vi "Ejercicio_14_daq_sensor.vi"() -> ()   [LabVIEW 2020]
panel:
  out "XY Graph":cluster{dbl[], dbl[]}[](graph)
  out "Waveform Chart":dynamicdata(graph)
  out "array":dbl[](array[numeric])
  out "array 2":dbl[](array[numeric])
  in  "stop":bool
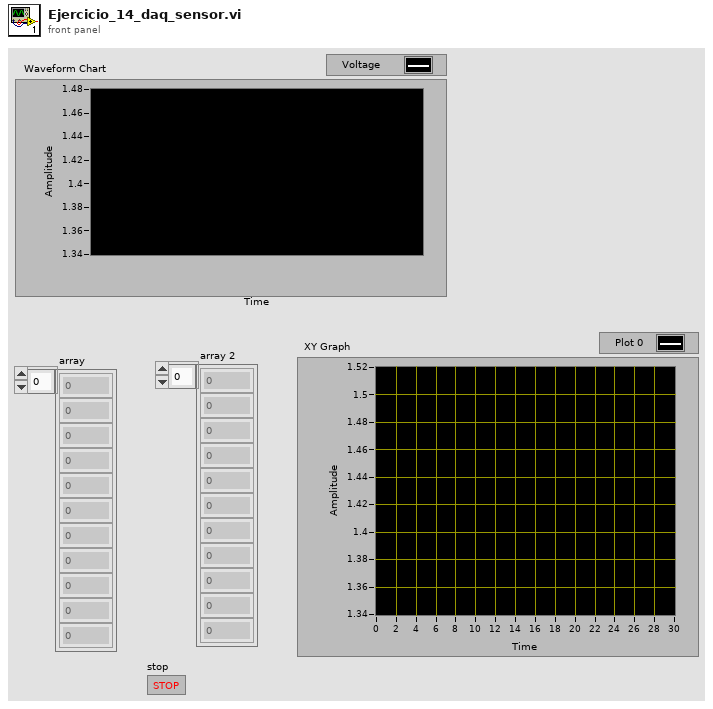
[diagram p1: front panel]
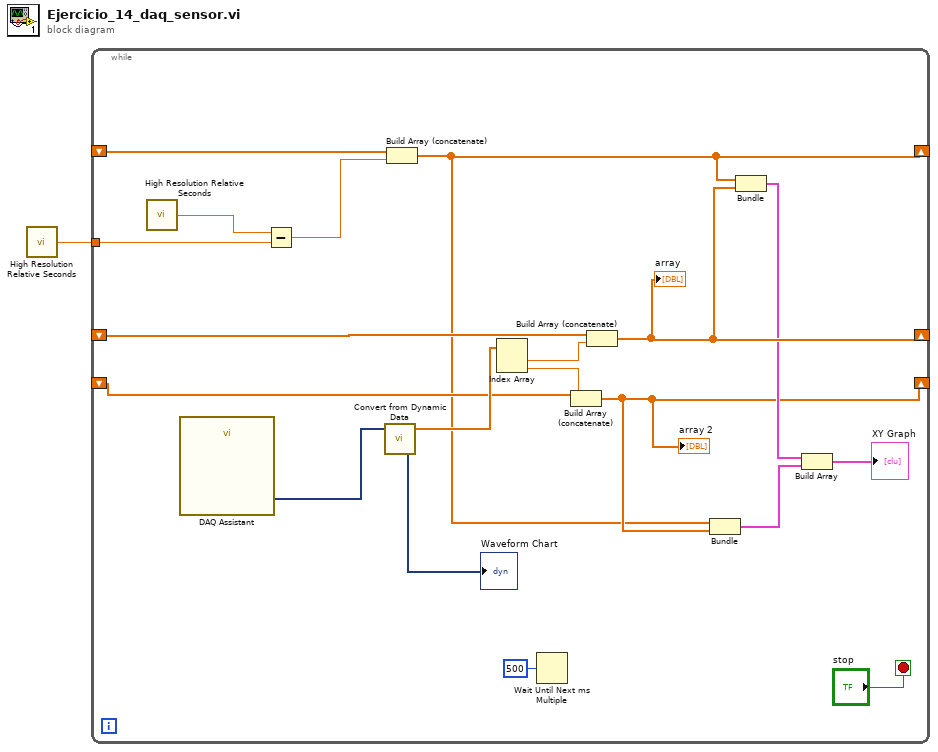
[diagram p0: block diagram]
diagram:
  n1 = call <vilib>:"High Resolution Relative Seconds.vi"() -> ("relative seconds"=w1:dbl)
  n2 = while {
    shift-right: [w8] -> _
    shift-left: _ -> [w15]
    shift-right: [w6] -> _
    shift-left: _ -> [w14]
    tunnel: w1 -> [w11]
    shift-right: [w5] -> _
    shift-left: _ -> [w9]
    stop <- "stop" stop-if-true
    n3 = call <vilib>:"High Resolution Relative Seconds.vi"() -> ("relative seconds"=w12:dbl)
    n4 = call "DAQ Assistant"() -> ("data"=w13:dynamicdata)  [unwired: 17 in, 2 out]
    "Waveform Chart" <- w13
    n5 = Subtract(x=w12, y=w11) -> (x-y=w10:dbl)
    n6 = call "Convert from Dynamic Data"("Dynamic Data Type"=w13) -> ("Array"=w18:dbl[])  [unwired: 3 in]
    n7 = Build Array (concatenate) "Build Array"(w9, w10) -> (w5:dbl[])
    n8 = Index Array "Index Array"(array=w18) -> (element #1=w16:dbl, element #2=w17:dbl)  [unwired: 2 in]
    n9 = Wait Until Next ms Multiple(millisecond multiple=u32 500) -> ()  [unwired: 1 out]
    n10 = Build Array (concatenate) "Build Array"(w14, w17) -> (w6:dbl[])
    "array 2" <- w6
    n11 = Build Array (concatenate) "Build Array"(w15, w16) -> (w8:dbl[])
    "array" <- w8
    n12 = Bundle "Bundle"(w5, w6) -> (w4:cluster{dbl[], dbl[]})  [unwired: 1 in]
    n13 = Bundle "Bundle"(w5, w8) -> (w7:cluster{dbl[], dbl[]})  [unwired: 1 in]
    n14 = Build Array "Build Array"(w7, w4) -> (→"XY Graph":cluster{dbl[], dbl[]}[])
  }
